vi "Wait for stop.vi"(1 "Port":T1={"P type"=0, "reference"="", " Terminator "="\r\n", "Timeout"=300} {"Timeout" step=10; "P type" items=["none", "RS-232C"]}, 3 "error in (no error)":errorcluster, 4 "wait for in pos":bool, 5 "Controller #":string) -> (9 "error out":errorcluster)   [LabVIEW 2015]
doc: "等待停止"
panel:
  out "new time":u32
  out "In position?":bool
  out "Moving?":bool
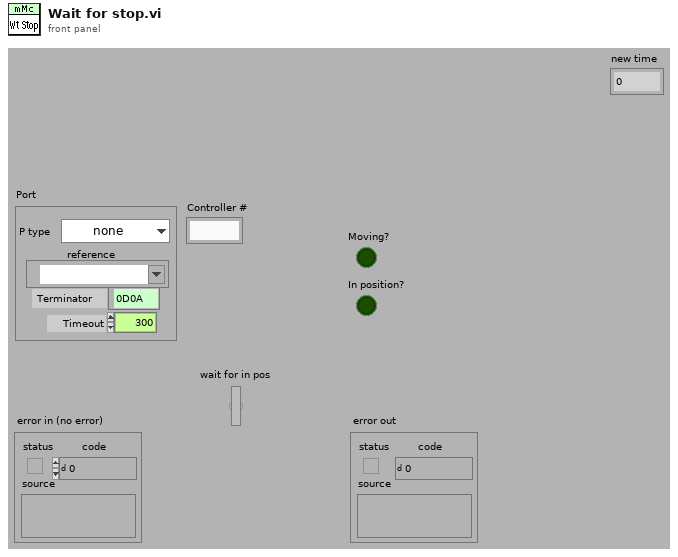
[diagram p1: front panel]
types:
  T1 = cluster{"P type":u16, "reference":refnum<visa-resource-name>, " Terminator ":string, "Timeout":i32}
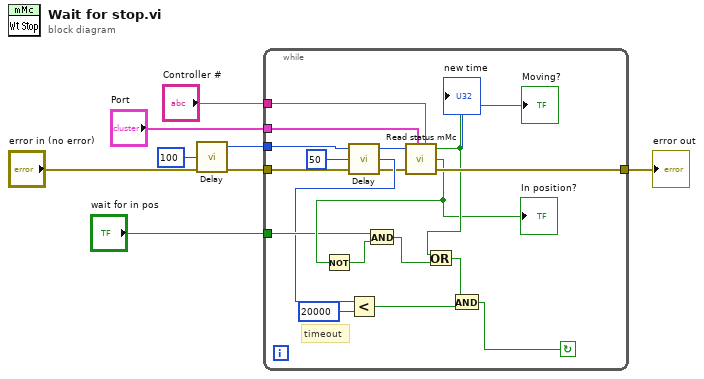
[diagram p0: block diagram]
diagram:
  n1 = call <instrlib>:"Delay.vi"("milliseconds to wait"=u32 100, "error in (no error)"="error in (no error)") -> ("new time"=w3:u32, "error out"=w1:errorcluster)  [unwired: 5 in, 1 out]
  n2 = while {
    tunnel: "Port" -> [w26]
    tunnel: "Controller #" -> [w25]
    tunnel: [w24] -> w6
    tunnel: "wait for in pos" -> [w19]
    tunnel: w3 -> [w9]
    tunnel: w1 -> [w11]
    stop <- w13 continue-if-true
    # "timeout"
    n3 = call <instrlib>:"Delay.vi"("old timer value"=w9, "milliseconds to wait"=u32 50, "error in (no error)"=w11) -> ("new time"=→"new time":u32, "elapsed time"=w17:u32, "error out"=w10:errorcluster)  [unwired: 4 in]
    n4 = Less?(x=w17, y=u32 20000) -> (x < y?=w15:bool)
    n5 = call <instrlib>:"Read status mMc.vi"("Port"=w26, "error in (no error)"=w10, "Controller #"=w25) -> ("Moving?"=w22:bool, "In position?"=w21:bool, "error out"=w24:errorcluster)  [unwired: 4 in]
    "Moving?" <- w22
    "In position?" <- w21
    n6 = Not(x=w21) -> (.not. x?=w18:bool)
    n7 = And(x=w19, y=w18) -> (x .and. y?=w20:bool)
    n8 = Or(x=w22, y=w20) -> (x .or. y?=w14:bool)
    n9 = And(x=w14, y=w15) -> (x .and. y?=w13:bool)
  }
  "error out" <- w6
